vi "HV Volt Monitor.vi"() -> (0 "Monitor":string[][](array[string])=[["Ch", "ISet", "VSet", "VMon", "SWVMax", "IMon", "RUp", "RDwn", "Status\nV6534PA"], ["0", "250.000uA", "1000.000V", "1.600V", "2000V", "0.000uA", "100Vps", "100Vps", "OFF\nV6534PA"], ["1", "250.000uA", "1500.000V", "0.100V", "2000V", "0.000uA", "100Vps", "100Vps", "OFF\nV6534PA"], ["2", "250.000uA", "1480.000V", "0.000V", "2000V", "0.000uA", "100Vps", "100Vps", "OFF\nV6534PA"], ["3", "250.000uA", "1200.000V", "1.400V", "2000V", "0.000uA", "100Vps", "100Vps", "OFF\nV6534PA"], ["4", "250.000uA", "1000.000V", "0.000V", "2000V", "0.000uA", "100Vps", "100Vps", "OFF\nV6534PA"], ["5", "250.000uA", "1000.000V", "0.000V", "2000V", "0.000uA", "100Vps", "100Vps", "OFF\nV6534PB"], ["0", "250.000uA", "1000.000V", "1.300V", "2000V", "0.000uA", "100Vps", "100Vps", "OFF\nV6534PB"], ["1", "250.000uA", "1000.000V", "0.000V", "2000V", "0.000uA", "100Vps", "100Vps", "OFF\nV6534PB"], ["2", "250.000uA", "100.000V", "0.000V", "2000V", "0.000uA", "100Vps", "100Vps", "OFF\nV6534PB"], ["3", "250.000uA", "100.000V", "1.300V", "2000V", "0.000uA", "100Vps", "100Vps", "OFF\nV6534PB"], ["4", "250.000uA", "100.000V", "0.000V", "2000V", "0.000uA", "100Vps", "100Vps", "OFF\nV6534PB"], ["5", "250.000uA", "100.000V", "0.000V", "2000V", "0.000uA", "100Vps", "100Vps", "OFF"]], 3 "Errors":string[](array[string]))   [LabVIEW 2018, in "HV QMH.lvlib"]
uses:
  HV QMH.lvlib
panel:
  # "- Creates array of values to monitor all parameters\n- Select channel and parameter to monitor individual values"
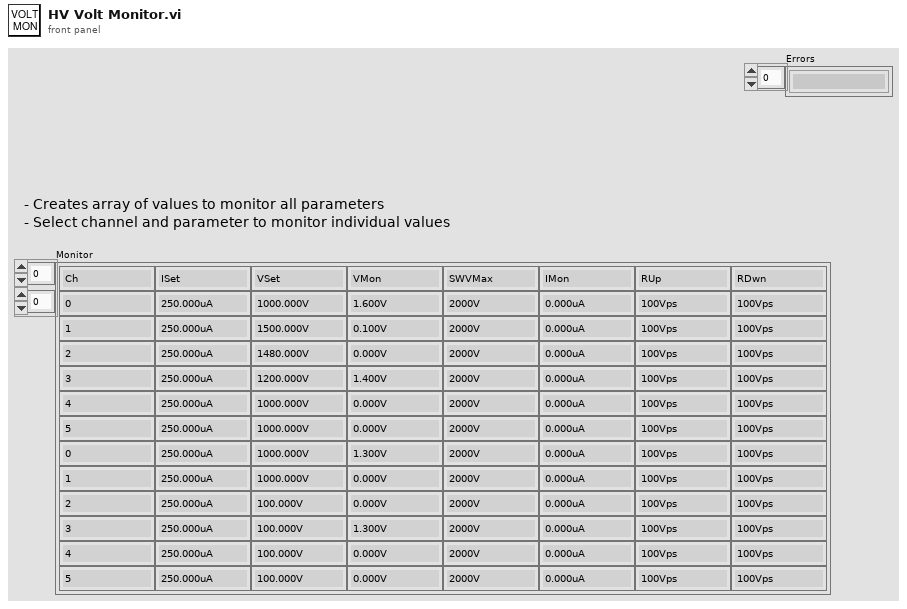
[diagram p1: front panel]
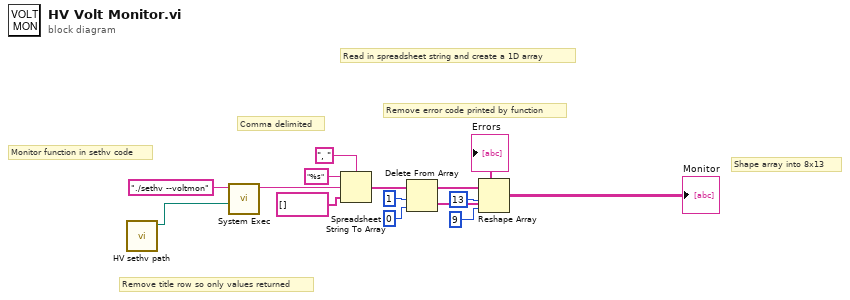
[diagram p0: block diagram]
diagram:
  # "Remove title row so only values returned"
  # "Shape array into 8x13"
  # "Remove error code printed by function"
  # "Monitor function in sethv code"
  # "Comma delimited"
  # "Read in spreadsheet string and create a 1D array"
  n1 = call "HV sethv path.vi"() -> ("sethv filepath"=w2:path)  [unwired: 11 in]
  n2 = call <vilib>:"System Exec.vi"("working directory"=w2, "command line"="./sethv --voltmon") -> ("standard output"=w13:string)  [unwired: 6 in, 3 out]
  n3 = Spreadsheet String To Array(delimiter (Tab)=", ", format string="%s", spreadsheet string=w13, array type (2D Dbl)=string[] []) -> (array=w10:string[])
  n4 = Delete From Array(array=w10, length=1, index=0) -> (deleted portion=→"Errors":string[], array with subset deleted=w5:string[])
  n5 = Reshape Array(w5, 13 ("dimension size"), 9 ("dimension size")) -> (→"Monitor":string[][])
